vi "TEMPLATE_Regular_NoReturn.vi"(8 "Error In":errorcluster, 11 "%TYPE% In":refnum<class "LQSerialData.lvclass">) -> (0 "Error Out":errorcluster, 3 "%TYPE% Out":refnum<class "LQSerialData.lvclass">)   [LabVIEW 2013, in "Template.lvlib" / "LQSerialData.lvclass"]
uses:
  LQSerialData.lvclass
  LQSerialData.lvclass/LQSerialData.ctl
  LQWidgetEngine/LQWidgetEngine.lvclass
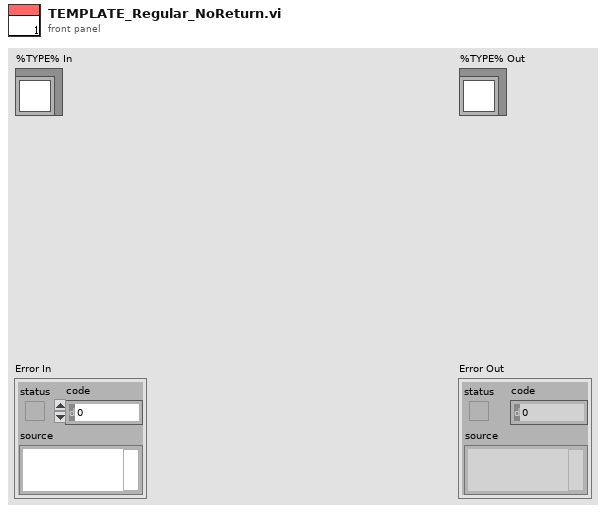
[diagram p1: front panel]
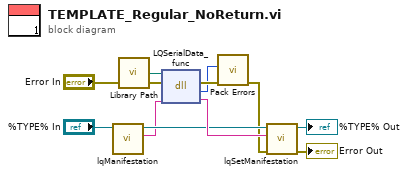
[diagram p0: block diagram]
diagram:
  n1 = call "lqManifestation.vi"("LQSerialData in"="%TYPE% In") -> ("Manifestation"=w6:string, "LQSerialData out"=w7:refnum<class "LQSerialData.lvclass">)  [unwired: 9 in]
  n2 = call "Library Path.vi"() -> ("Library Path"=w5:path)
  n3 = dll-call lib="?" fn="LQSerialData_func"(path in=w5, error in="Error In", "_instance"=w6) -> (error out=w4:errorcluster, "errorCode"=w3:i32, "_instance"=w9:string)  [unwired: 1 in, 1 out]
  n4 = call "Pack Errors.vi"("Error In"=w4, "Error Code"=w3) -> ("Error Out"=w2:errorcluster)  [unwired: 9 in]
  n5 = call "lqSetManifestation.vi"("Error In"=w2, "Manifestation"=w9, "LQSerialData in"=w7) -> ("Error Out"=→"Error Out":errorcluster, "LQSerialData out"=→"%TYPE% Out":refnum<class "LQSerialData.lvclass">)  [unwired: 7 in]
